vi "(SubVI) Wang 97 Tether Calibration.vi"(0 "Set lower foce offset?":bool, 4 "X=T\nY=F":bool=TRUE, 5 "QPD signal":dbl[](array[numeric]), 6 "Stage Position":dbl[](array[numeric]), 7 "Fitting Cluster":T1={"cr (um)"=0.0, "yr (V)"=0.0, "trap height(nm)"=300.0, "bead radius(nm)"=515.0, "Length offset"=400.0, "Upper Force(pN)"=5.0, "cr shift (nm)"=0.0, "yr shift (mV)"=0.0, "LaserPower (mW)"=20.0, "conversion factor (V/um)"=0.0, "Stiffness (pN/nm)"=0.0, "xDNA cut outside"=3000.0, "Lower Force(pN)"=5.0, "c for zbd"=0.0}) -> (1 "Force":dbl[](array[numeric]), 2 "xDNA":dbl[](array[numeric]), 3 "output cluster":T1={"cr (um)"=0.0, "yr (V)"=0.0, "trap height(nm)"=0.0, "bead radius(nm)"=520.0, "Length offset"=0.0, "Upper Force(pN)"=0.0, "cr shift (nm)"=0.0, "yr shift (mV)"=0.0, "LaserPower (mW)"=0.0, "conversion factor (V/um)"=0.0, "Stiffness (pN/nm)"=0.0, "xDNA cut outside"=0.0, "Lower Force(pN)"=5.0, "c for zbd"=0.0})   [LabVIEW 2014]
uses:
  WLC-Fitting Cluster.ctl
panel:
  out "XY Graph 2":cluster{"zbd (nm)":dbl[], "Force":dbl[]}(graph)
  out "XY Graph":cluster{"zbd (nm)":dbl[], "Force":dbl[]}(graph)
  out "Waveform Graph":dbl[](graph)
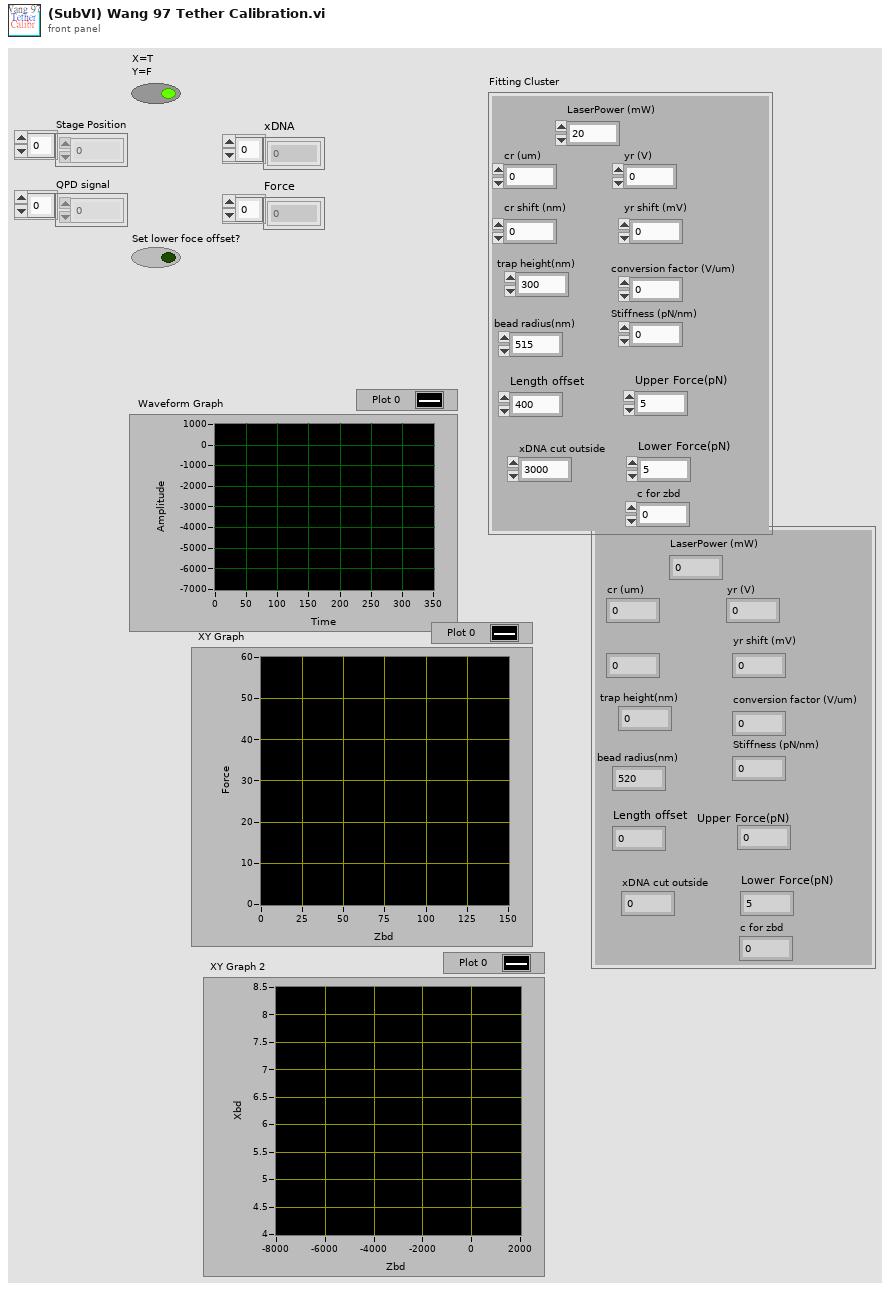
[diagram p1: front panel]
types:
  T1 = typedef "WLC-Fitting Cluster.ctl" = cluster{"cr (um)":dbl, "yr (V)":dbl, "trap height(nm)":dbl, "bead radius(nm)":dbl, "Length offset":dbl, "Upper Force(pN)":dbl, "cr shift (nm)":dbl, "yr shift (mV)":dbl, "LaserPower (mW)":dbl, "conversion factor (V/um)":dbl, "Stiffness (pN/nm)":dbl, "xDNA cut outside":dbl, "Lower Force(pN)":dbl, "c for zbd":dbl}
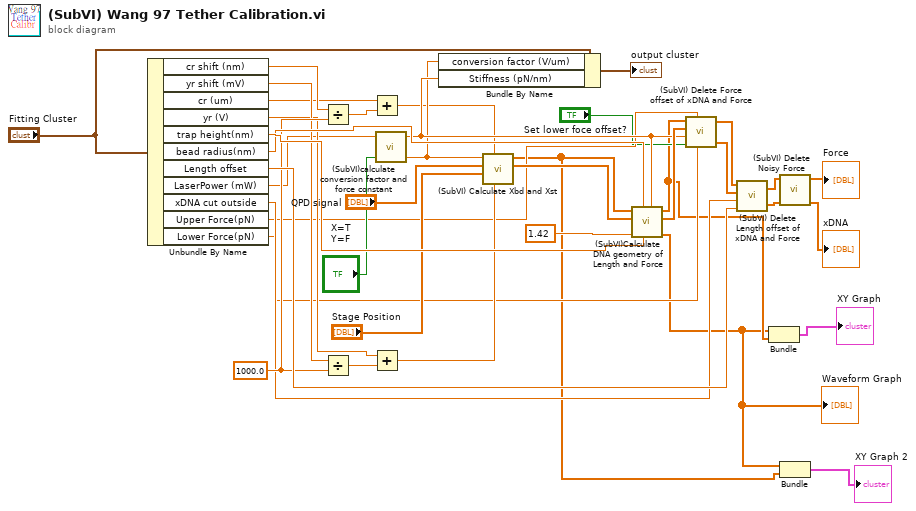
[diagram p0: block diagram]
diagram:
  w32 = 1000.0 ("y")
  n1 = Unbundle By Name("Fitting Cluster") -> ("cr shift (nm)"=w31:dbl, "yr shift (mV)"=w30:dbl, "cr (um)"=w28:dbl, "yr (V)"=w26:dbl, "trap height(nm)"=w35:dbl, "bead radius(nm)"=w34:dbl, "Length offset"=w33:dbl, "LaserPower (mW)"=w24:dbl, "xDNA cut outside"=w9:dbl, "Upper Force(pN)"=w8:dbl, "Lower Force(pN)"=w7:dbl)
  n2 = Divide(x=w31, y=w32) -> (x/y=w29:dbl)
  n3 = Divide(x=w30, y=w32) -> (x/y=w27:dbl)
  n4 = Add(x=w28, y=w29) -> (x+y=w20:dbl)
  n5 = Add(x=w26, y=w27) -> (x+y=w25:dbl)
  n6 = call "(SubVI)calculate conversion factor and force constant.vi"("X=T\nY=F"="X=T\nY=F", "laser power (mW)"=w24) -> ("conversion factor (V/um)"=w22:dbl, "force constant (pN/nm)"=w23:dbl)  [unwired: 2 in]
  n7 = Bundle By Name(cluster="Fitting Cluster", "conversion factor (V/um)"=w22, "Stiffness (pN/nm)"=w23) -> (→"output cluster":T1)
  n8 = call "(SubVI) Calculate Xbd and Xst.vi"("yr"=w25, "cr"=w20, "Stage Position"="Stage Position", "QPD signal"="QPD signal", "conversion factor (V/um)"=w22) -> ("Xst"=w17:dbl[], "Xbd"=w2:dbl[])  [unwired: 5 in]
  n9 = call "(SubVI)Calculate DNA geometry of Length and Force.vi"("Force constant (pN/nm)"=w23, "trap height(nm)"=w35, "bead radius(nm)"=w34, "Focal shift factor"=1.42, "Xst"=w17, "Xbd"=w2) -> ("zbd (nm)"=w1:dbl[], "xDNA"=w38:dbl[], "Force"=w4:dbl[])  [unwired: 3 in]
  "Waveform Graph" <- w1
  n10 = call "(SubVI) Delete Force offset of xDNA and Force.vi"("Force"=w4, "Upper Force (pN)"=w8, "xDNA"=w38, "force constant"=w23, "Lower Force (pN)"=w7, "Set lower foce offset?"="Set lower foce offset?") -> ("cut-full Force"=w37:dbl[], "cut-full xDNA"=w36:dbl[])  [unwired: 1 in]
  n11 = call "(SubVI) Delete Length offset of xDNA and Force.vi"("Length offset"=w33, "xDNA cut outside (nm)"=w9, "xDNA"=w36, "Force"=w37) -> ("cut-full xDNA"=w14:dbl[], "cut-full Force"=w15:dbl[])
  n12 = Bundle("zbd (nm)"=w1, "Force"=w4) -> (→"XY Graph":cluster{"zbd (nm)":dbl[], "Force":dbl[]})  [unwired: 1 in]
  n13 = call "(SubVI) Delete Noisy Force.vi"("xDNA"=w14, "Force"=w15) -> ("xDNA-cut"=→"xDNA":dbl[], "Force-cut"=→"Force":dbl[])  [unwired: 4 in]
  n14 = Bundle("zbd (nm)"=w1, "Xbd"=w2) -> (→"XY Graph 2":cluster{"zbd (nm)":dbl[], "Xbd":dbl[]})  [unwired: 1 in]
